vi "NI9234_SUB-VI_EngineACQ.vi"(8 "error in":errorcluster) -> (0 "error out":errorcluster)   [LabVIEW 2020]
uses:
  TYPEDEF/NI9234_TD_MethodNI9234.ctl
  RPA_BACKDRIVE/GUI/SUBVI/TYPEDEF/ClusterSaveData.ctl
  RPA_BACKDRIVE/GUI/SUBVI/TYPEDEF/SaveData.ctl
  TYPEDEF/NI9234_TD_Method_Queue.ctl
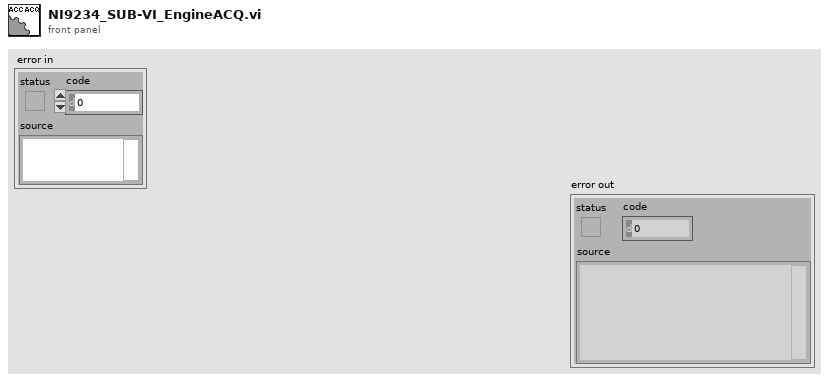
[diagram p1: front panel]
types:
  T1 = typedef "NI9234_TD_Method_Queue.ctl" = enum16{"NO_OP", "CREATE", "POPULATE", "FLUSH", "DESTROY", "DEL_ELEM", "GET_STATUS"}
  T2 = typedef "SaveData.ctl" = enum16{"NO_OP", "FUNZIONE", "INVIA_DATI", "RILETTURA"}
  T3 = typedef "ClusterSaveData.ctl" = cluster{"VariantValue":variant, "SaveData":T2}
  T4 = typedef "NI9234_TD_MethodNI9234.ctl" = enum16{"NO_OP", "INIT", "SET", "GET", "CLOSE"}
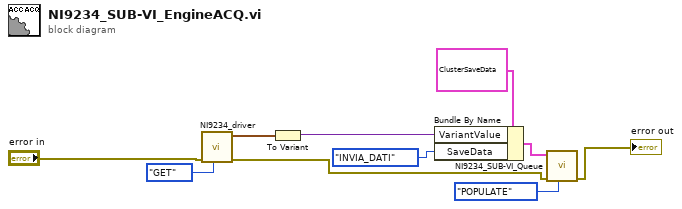
[diagram p0: block diagram]
diagram:
  n1 = call "NI9234_driver.vi"("Method NI9205"=NI9234_TD_MethodNI9234."GET", "error in"="error in") -> ("error out"=w2:errorcluster, "data"=w3:waveform(dbl)[])  [unwired: 6 in, 2 out]
  n2 = To Variant(anything=w3) -> (Variant=w6:variant)
  n3 = Bundle By Name(cluster=T3 {"VariantValue"=variant, "SaveData"=enum."NO_OP"} ("Cluster_SaveData"), "VariantValue"=w6, "SaveData"=SaveData."INVIA_DATI") -> (w5:T3)
  n4 = call "NI9234_SUB-VI_Queue.vi"("Method"=NI9234_TD_Method_Queue."POPULATE", "error in (no error)"=w2, "Cluster_SaveData"=w5) -> ("error out"=→"error out":errorcluster)  [unwired: 6 in, 2 out]
